vi "Close.vi"(8 "error in (no error)":errorcluster, 11 "VISA resource name":refnum<visa-resource-name>) -> (0 "error out":errorcluster)   [LabVIEW 2018]
doc: "Performs an instrument error query before terminating the software connection to the instrument."
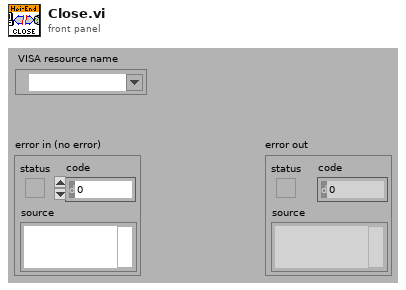
[diagram p1: front panel]
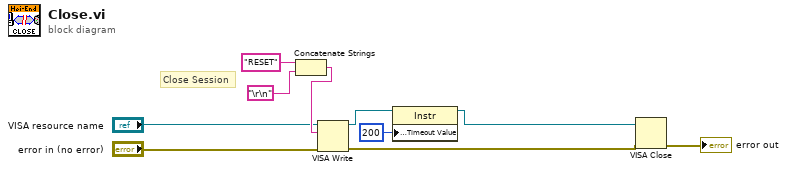
[diagram p0: block diagram]
diagram:
  # "Close Session"
  n1 = Concatenate Strings("RESET" ("format string"), "\r\n") -> (w5:string)
  n2 = VISA Write(VISA resource name="VISA resource name", write buffer=w5, error in (no error)="error in (no error)") -> (VISA resource name out=w8:refnum<visa-resource-name>, error out=w3:errorcluster)  [unwired: 1 out]
  n3 = property class="Instr"(reference=w8, "General Settings:Timeout Value"=u32 200) -> (reference out=w4:refnum<visa-resource-name>)  [unwired: 1 in, 1 out]
  n4 = VISA Close(VISA resource name=w4, error in (no error)=w3) -> (error out=→"error out":errorcluster)
